vi "Periodic Tasks.vi"(8 "error in":errorcluster) -> ()   [LabVIEW 2019]
doc: "This VI runs in parallel to other tasks. It can contain as many user-defined periodic loops as you need. These can carry out PID or other sorts of timed response."
uses:
  <vilib>/Rock Robotics/WPI/Relay/WPI_RelayValue.ctl
  <vilib>/Rock Robotics/WPI/Utilities/WPI_GetSetVariantRefNum.vi
  Robot Global Data.vi
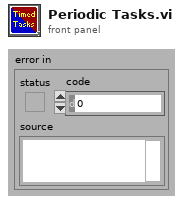
[diagram p1: front panel]
types:
  T1 = typedef "WPI_RelayDevRef.ctl" = cluster{"DevStatus":errorcluster, "Relay Channel":T2, "Relay Direction":T3}
  T2 = typedef "FPGA_DIORelayChannel.ctl" = enum8{"Relay 0", "Relay 1", "Relay 2", "Relay 3", "Invalid"}
  T3 = typedef "WPI_RelayDirection.ctl" = enum16{"Both directions", "Forward only", "Reverse only"}
  T4 = typedef "WPI_RelayValue.ctl" = enum16{"Off", "On", "Forward", "Reverse"}
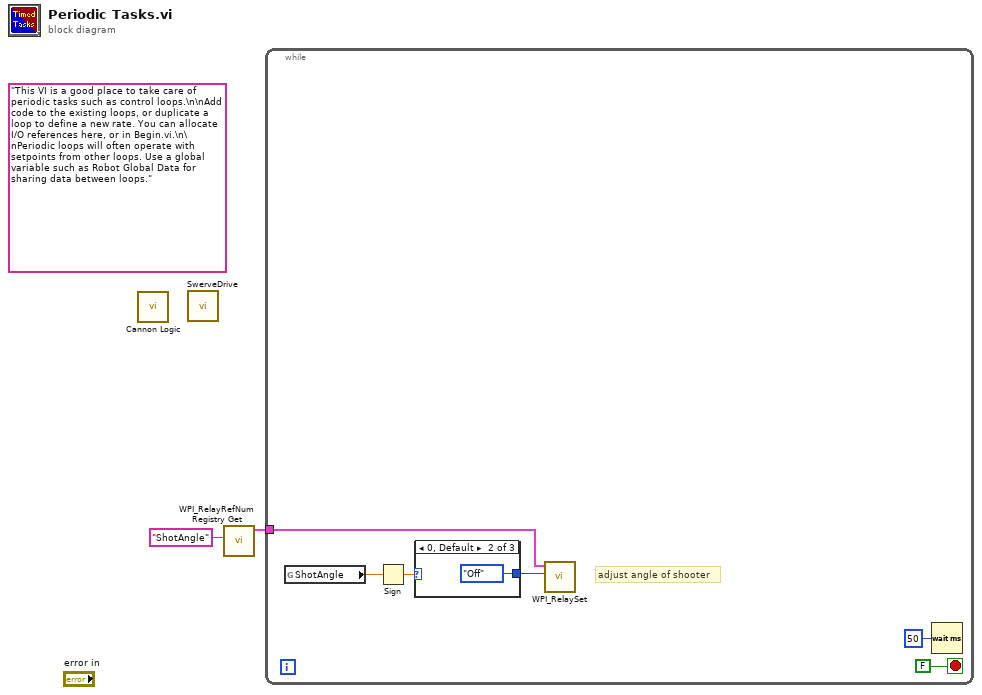
[diagram p0: block diagram]
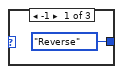
[diagram p2: hidden frame]
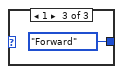
[diagram p3: hidden frame]
diagram:
  (unwired) "This VI is a good place to take care of periodic tasks such as control loops.\n\nAdd code to the existing loops, or duplicate a loop to define a new rate. You can allocate I/O references here, or in Begin.vi.\n\nPeriodic loops will often operate with setpoints from other loops. Use a global variable such as Robot Global Data for sharing data between loops."
  n1 = call "Cannon Logic.vi"() -> ()  [unwired: 12 in]
  n2 = call "SwerveDrive.vi"() -> ()  [unwired: 12 in]
  n3 = call <vilib>:"WPI_RelayRefNum Registry Get.vi"("refnum name"="ShotAngle") -> ("RelayDevRef"=w1:T1)  [unwired: 9 in, 1 out]
  n4 = while {
    tunnel: w1 -> [w6]
    stop <- FALSE stop-if-true
    # "adjust angle of shooter"
    n5 = global read "Robot Global Data.vi" "ShotAngle"() -> (w3:dbl)
    n6 = Sign(1:w3) -> (0:w4:dbl)
    n7 = case shown="0, Default" w4 {
      tunnel: [WPI_RelayValue."Reverse" ("YawAdjustment") WPI_RelayValue."Off" ("YawAdjustment") WPI_RelayValue."Forward" ("YawAdjustment")] -> w5
      frame -1 {
      }
      frame 0, Default {
      }
      frame 1 {
      }
    }
    n8 = call <vilib>:"WPI_RelaySet.vi"("RelayValue"=w5, "RelayDevRef"=w6) -> ()  [unwired: 8 in, 2 out]
    n9 = Wait (ms)(milliseconds to wait=u32 50) -> ()  [unwired: 1 out]
  }
